vi "Save Device Info.vi"(8 "error in":errorcluster, 10 "Array of Device Info":T1, 11 "File Path":path) -> (0 "error out":errorcluster)   [LabVIEW 2016]
uses:
  Array Device Info.ctl
  Device Info.ctl
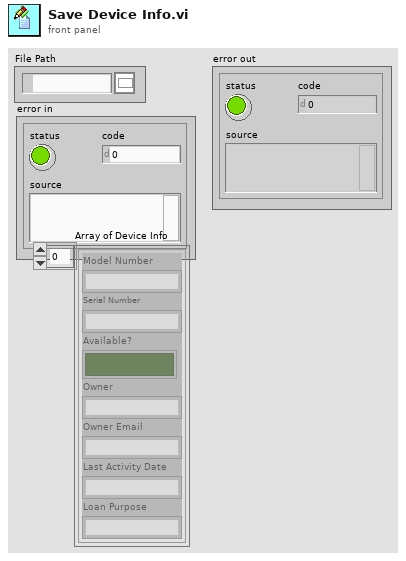
[diagram p1: front panel]
types:
  T1 = typedef "Array Device Info.ctl" = T2[]
  T2 = typedef "Device Info.ctl" = cluster{"Model Number":string, "Serial Number":string, "Available?":bool, "Owner":string, "Owner Email":string, "Last Activity Date":string, "Loan Purpose":string}
  T3 = enum16{"open", "replace", "create", "open or create", "replace or create", "replace or create with confirmation"}
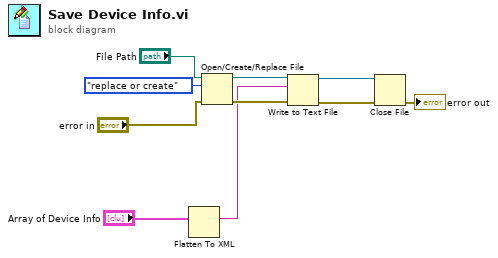
[diagram p0: block diagram]
diagram:
  n1 = Flatten To XML(anything="Array of Device Info") -> (xml string=w2:string)
  n2 = Open/Create/Replace File(file path (use dialog)="File Path", error in="error in", operation (0:open)=T3."replace or create") -> (refnum out=w10:refnum<file>, error out=w8:errorcluster)  [unwired: 3 in, 1 out]
  n3 = Write to Text File(file (use dialog)=w10, text=w2, error in=w8) -> (refnum out=w9:refnum<file>, error out=w7:errorcluster)  [unwired: 1 in, 1 out]
  n4 = Close File(refnum=w9, error in=w7) -> (error out=→"error out":errorcluster)  [unwired: 1 out]
